vi "DtOLRead.vi"   [LabVIEW 2016]
doc: "Reads samples from the virtual channels of a task you specify. This VI implicitly starts the task; therefore, you do not need to call the OLStart VI when using this VI. \n\nThe instances of this polymorphic VI specify the format of the data to return, whether to read a single channel or multiple channels, and whether to read a single sample or multiple samples."
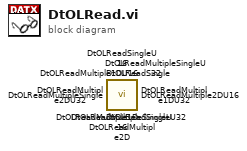
[diagram p0: block diagram]
diagram:
  n1 = call <userlib>:"DtOLReadMultipleSingleU16.vi"() -> ()  [unwired: 7 in, 5 out]
  n2 = call <userlib>:"DtOLReadMultipleSingleU32.vi"() -> ()  [unwired: 7 in, 5 out]
  n3 = call <userlib>:"DtOLReadMultipleSingle.vi"() -> ()  [unwired: 7 in, 5 out]
  n4 = call <userlib>:"DtOLReadMultiple2DU16.vi"() -> ()  [unwired: 7 in, 5 out]
  n5 = call <userlib>:"DtOLReadMultiple1DU16.vi"() -> ()  [unwired: 8 in, 4 out]
  n6 = call <userlib>:"DtOLReadSingleU16.vi"() -> ()  [unwired: 9 in, 3 out]
  n7 = call <userlib>:"DtOLReadMultiple2DU32.vi"() -> ()  [unwired: 7 in, 5 out]
  n8 = call <userlib>:"DtOLReadMultiple1DU32.vi"() -> ()  [unwired: 8 in, 4 out]
  n9 = call <userlib>:"DtOLReadSingleU32.vi"() -> ()  [unwired: 9 in, 3 out]
  n10 = call <userlib>:"DtOLReadMultiple2D.vi"() -> ()  [unwired: 7 in, 5 out]
  n11 = call <userlib>:"DtOLReadMultiple1D.vi"() -> ()  [unwired: 8 in, 4 out]
  n12 = call <userlib>:"DtOLReadSingle.vi"() -> ()  [unwired: 9 in, 3 out]
